vi "check cluster field names.vi"(8 "error in (no error)":errorcluster, 11 "cluster in":variant) -> (0 "error out":errorcluster)   [LabVIEW 2018, in "LV-Julia_ZMQ-Roundtrip_lib.lvlib"]
uses:
  LV-Julia_ZMQ-Roundtrip_lib.lvlib
  <vilib>/Utility/Data Type/NI_Data Type.lvlib
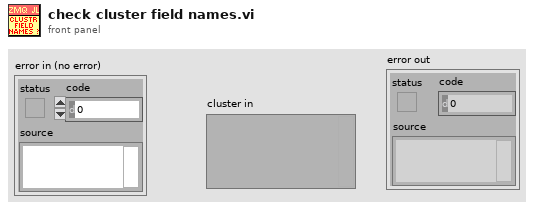
[diagram p1: front panel]
types:
  T1 = typedef "NI_Data Type.lvlib/Data Type.ctl" = enum8{"Invalid Type", "Void", "I8", "I16", "I32", "I64", "U8", "U16", "U32", "U64", "Single Float", "Double Float", "Extended Float", "Single Complex", "Double Complex", "Extended Complex", "Enum U8", "Enum U16", "Enum U32", "Enum U64", "Single Float With Unit", "Double Float With Unit", "Extended Float With Unit", "Single Complex with Unit", "Double Complex with Unit", "Extended Complex with Unit", "Boolean", "String", "Path", "Picture", "Tag", "Array", "Cluster", "Variant", "LV Variant", "Waveform", "Timestamp", "Digital Waveform", "Digital Data", "ExpressData", "Refnum", "External Data", "VI", "Poly VI", "LabVIEW Class Instance", "Fixed Point"}
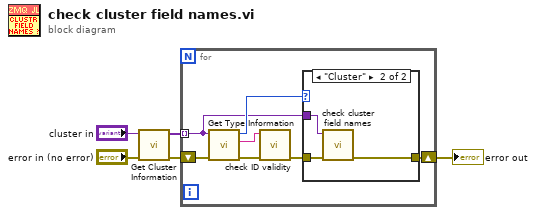
[diagram p0: block diagram]
diagram:
  n1 = call <vilib>:"Get Cluster Information.vi"("error in (no error)"="error in (no error)", "Variant"="cluster in") -> ("error out"=w2:errorcluster, "Cluster Elements"=w3:variant[])  [unwired: 8 in]
  n2 = for {
    tunnel: w3 -> [w6] mode=indexing
    shift-right: [w8] -> w1
    shift-left: w2 -> [w12]
    n3 = call <vilib>:"Get Type Information.vi"("error in (no error)"=w12, "Variant"=w6) -> ("error out"=w11:errorcluster, "Name"=w10:string, "Type"=w7:T1)  [unwired: 5 in, 2 out]
    n4 = call "check ID validity.vi"("error in (no error)"=w11, "ID in"=w10) -> ("error out"=w9:errorcluster)  [unwired: 8 in, 1 out]
    n5 = case shown="\"Cluster\"" w7 {
      tunnel: [w13 w15] -> w8
      tunnel: w9 -> [w13 w16]
      tunnel: w6 -> [_ w14]
      frame "Invalid Type", Default {
      }
      frame "Cluster" {
        n6 = call "check cluster field names.vi"("error in (no error)"=w16, "cluster in"=w14) -> ("error out"=w15:errorcluster)  [unwired: 9 in]
      }
    }
  }
  "error out" <- w1
